vi "Initialize Settings.vi"(8 "error in (no error)":errorcluster, 11 "Sensor & Control in":refnum<class "Sensor.lvclass">) -> (0 "error out":errorcluster, 1 "Sampling Interval 2":i32, 2 "VISA out":refnum<visa-resource-name>, 3 "Sensor & Control out":refnum<class "Sensor.lvclass">)   [LabVIEW 2013, in "Sensor.lvib.lvlib" / "Sensor.lvclass"]
uses:
  Sensor.lvclass
  PluginInterface/PluginInterface.lvlibp/PluginInterfaceClass/Read Name.vi
panel:
  in  "Sampling Interval":i32
  in  "String":string
  in  "Button":bool
  in  "VISA in":refnum<visa-resource-name>
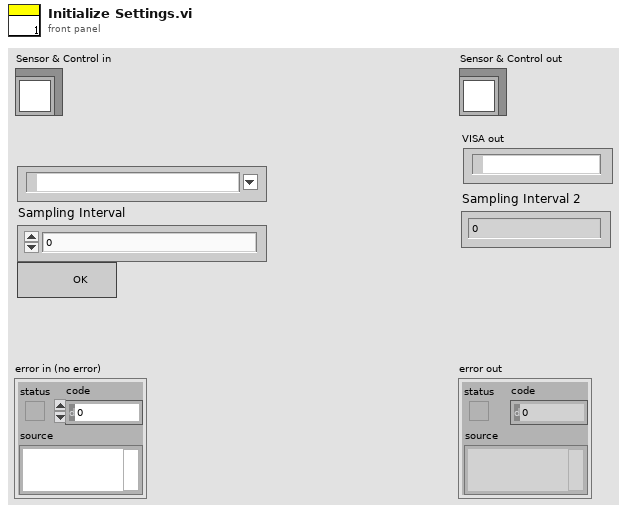
[diagram p1: front panel]
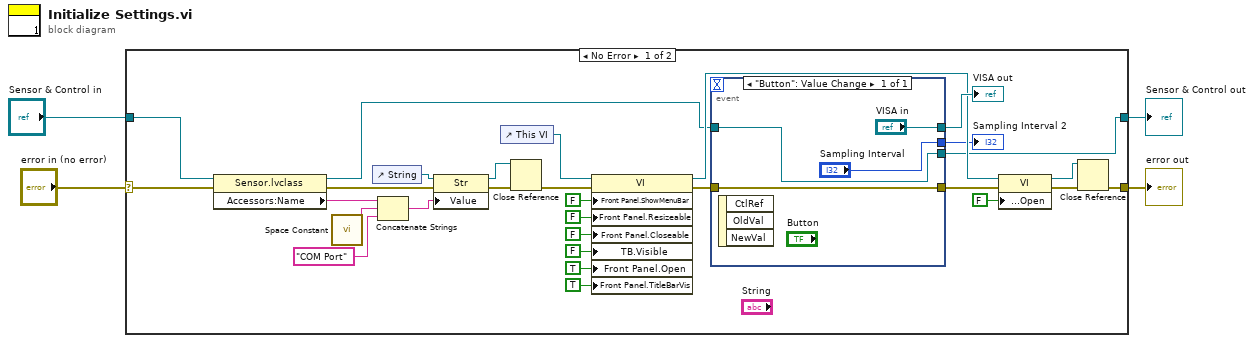
[diagram p0: block diagram]
diagram:
  n1 = case shown="No Error" "error in (no error)" {
    selector: "error in (no error)" -> [w9 w39]
    tunnel: [w19 w39] -> w3
    tunnel: [w18 w38] -> w1
    tunnel: "Sensor & Control in" -> [w5 w38]
    frame No Error {
      n2 = property class="Sensor.lvclass"(reference=w5, error in=w9) -> (reference out=w8:refnum<class "Sensor.lvclass">, error out=w7:errorcluster, "Accessors:Name"=w6:string)
      n3 = call <vilib>:"Space Constant.vi"() -> ("String"=w10:string)
      n4 = control-ref of="String"() -> (w14:refnum<vi>)
      n5 = Concatenate Strings(w6, w10, "COM Port" ("string")) -> (w17:string)
      n6 = property class="Str"(reference=w14, error in=w7, "Value"=w17) -> (reference out=w16:refnum<vi>, error out=w15:errorcluster)
      n7 = control-ref of="This VI"() -> (w32:refnum<vi>)
      n8 = Close Reference(reference=w16, error in (no error)=w15) -> (error out=w13:errorcluster)
      n9 = property class="VI"(reference=w32, error in=w13, "Front Panel.ShowMenuBar"=FALSE ("Front Panel Window:Show Menu Bar"), "Front Panel.Resizeable"=FALSE ("Front Panel Window:Resizable"), "Front Panel.Closeable"=FALSE ("Front Panel Window:Closeable"), "TB.Visible"=FALSE ("Tool Bar:Visible"), "Front Panel.Open"=TRUE ("Front Panel Window:Open"), "Front Panel.TitleBarVis"=TRUE ("Front Panel Window:Title Bar Visible")) -> (reference out=w21:refnum<vi>, error out=w25:errorcluster)
      n10 = event shown="[0] \"Button\": Value Change" {
        selector: _ -> [_]
        dyn-events: _ -> [_]
        timeout: _ -> [_]
        tunnel: w25 -> [w36]
        tunnel: [w36] -> w20
        tunnel: ["VISA in"] -> w33
        tunnel: w8 -> [w35]
        tunnel: [w35] -> w18
        tunnel: ["Sampling Interval"] -> w12
        event "Button": Value Change {
          n11 = event-data() -> ()  [unwired: 1 in, 3 out]
        }
      }
      "VISA out" <- w33
      "Sampling Interval 2" <- w12
      n12 = property class="VI"(reference=w21, error in=w20, "Front Panel.Open"=FALSE ("Front Panel Window:Open")) -> (reference out=w24:refnum<vi>, error out=w23:errorcluster)
      n13 = Close Reference(reference=w24, error in (no error)=w23) -> (error out=w19:errorcluster)
    }
    frame Error {
    }
  }
  "error out" <- w3
  "Sensor & Control out" <- w1
